vi "Destructor.vi"(8 "error in":errorcluster, 11 "OperationRun":refnum<class "OperationRun.lvclass">) -> (0 "error out":errorcluster)   [LabVIEW 2021, in "ProligentXMLGenerator.lvlib" / "OperationRun.lvclass"]
uses:
  OperationRun.lvclass
  OperationRun.lvclass/OperationRun.ctl
  SequenceRun/SequenceRun/SequenceRun.lvclass
  Model/CustomData/CustomData.lvclass
  Model/Characteristic/Characteristic.lvclass
  Model/Document/Document.lvclass
  Failure/FailureReference/FailureReference.lvclass
  SequenceRun/SequenceRunReference/SequenceRunReference.lvclass
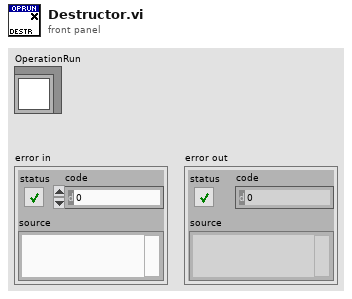
[diagram p1: front panel]
types:
  T1 = typedef "ProligentXMLGenerator.lvlib/OperationRun.lvclass/Data.ctl" = cluster{"Name":string, "Characteristics":refnum<class "Characteristic.lvclass">[], "Documents":refnum<class "Document.lvclass">[], "SequenceRuns":refnum<class "SequenceRun.lvclass">[], "FailureReferences":refnum<class "FailureReference.lvclass">[], "SequenceRunReferences":refnum<class "SequenceRunReference.lvclass">[], "CustomData":refnum<class "CustomData.lvclass">, "OperationRunId":refnum<class "Guid.lvclass">, "ProcessFullName":refnum<class "ProcessFullName.lvclass">, "ProcessVersion":refnum<class "NonEmptyString_64.lvclass">, "OperationName":refnum<class "NonEmptyString_65.lvclass">, "StationFullName":refnum<class "FullName.lvclass">, "User":refnum<class "NonEmptyString_255.lvclass">, "CallingOperationRunId":refnum<class "Guid.lvclass">, "OperationStatus":refnum<class "ExecutionStatus.lvclass">, "OperationRunStartTime":refnum<class "DateTime.lvclass">, "OperationRunEndTime":refnum<class "DateTime.lvclass">, "TimeZoneInfoId":string}
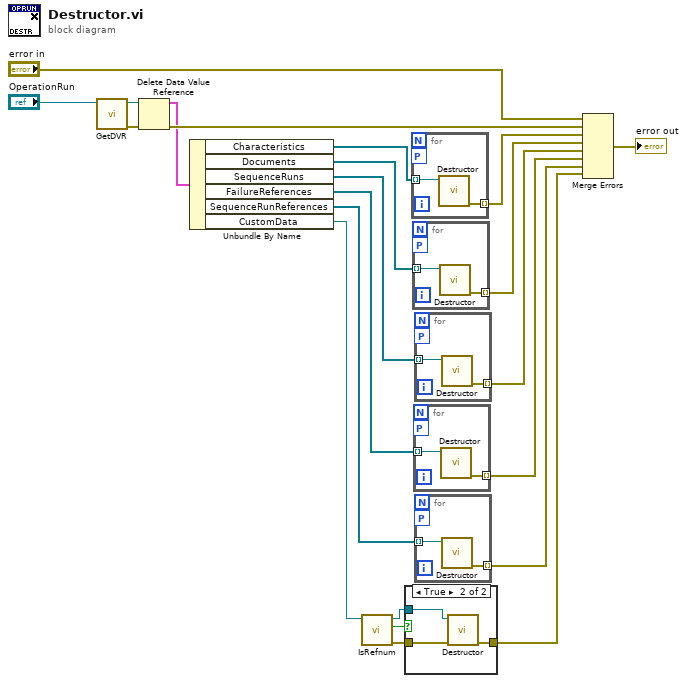
[diagram p0: block diagram]
diagram:
  n1 = call "GetDVR.vi"("OperationRun"="OperationRun") -> ("error out"=w19:errorcluster, "DVRReference"=w20:refnum<data-value>)  [unwired: 9 in]
  n2 = Delete Data Value Reference(data value reference=w20, error in=w19) -> (data value=w16:T1, error out=w17:errorcluster)
  n3 = Unbundle By Name(w16) -> ("Characteristics"=w15:refnum<class "Characteristic.lvclass">[], "Documents"=w13:refnum<class "Document.lvclass">[], "SequenceRuns"=w12:refnum<class "SequenceRun.lvclass">[], "FailureReferences"=w7:refnum<class "FailureReference.lvclass">[], "SequenceRunReferences"=w6:refnum<class "SequenceRunReference.lvclass">[], "CustomData"=w1:refnum<class "CustomData.lvclass">)
  n4 = call "IsRefnum.vi"("CustomDataType in"=w1) -> ("error out"=w3:errorcluster, "IsRefnum"=w5:bool, "CustomDataType out"=w4:refnum<class "CustomData.lvclass">)  [unwired: 8 in]
  n5 = case shown="True" w5 {
    tunnel: w4 -> [_ w26]
    tunnel: w3 -> [w23 w25]
    tunnel: [w23 w24] -> w2
    frame False {
    }
    frame True {
      n6 = call "Destructor.vi"("error in"=w25, "CustomDataType"=w26) -> ("error out"=w24:errorcluster)  [unwired: 9 in]
    }
  }
  n7 = for {
    tunnel: w15 -> [w28] mode=indexing
    tunnel: [w27] -> w14 mode=indexing
    workers-P: _ -> [_]
    n8 = call "Destructor.vi"("Document in"=w28) -> ("error out"=w27:errorcluster)  [unwired: 10 in]
  }
  n9 = for {
    tunnel: w13 -> [w30] mode=indexing
    tunnel: [w29] -> w11 mode=indexing
    workers-P: _ -> [_]
    n10 = call "Destructor.vi"("Document in"=w30) -> ("error out"=w29:errorcluster)  [unwired: 10 in]
  }
  n11 = for {
    tunnel: w7 -> [w32] mode=indexing
    tunnel: [w31] -> w9 mode=indexing
    workers-P: _ -> [_]
    n12 = call "Destructor.vi"("FailureReference in"=w32) -> ("error out"=w31:errorcluster)  [unwired: 10 in]
  }
  n13 = for {
    tunnel: w12 -> [w34] mode=indexing
    tunnel: [w33] -> w10 mode=indexing
    workers-P: _ -> [_]
    n14 = call "Destructor.vi"("SequenceRun"=w34) -> ("error out"=w33:errorcluster)  [unwired: 10 in]
  }
  n15 = for {
    tunnel: w6 -> [w36] mode=indexing
    tunnel: [w35] -> w8 mode=indexing
    workers-P: _ -> [_]
    n16 = call "Destructor.vi"("SequenceRunReference in"=w36) -> ("error out"=w35:errorcluster)  [unwired: 10 in]
  }
  n17 = Merge Errors("error in", w17, w14, w11, w10, w9, w8, w2) -> (→"error out":errorcluster)
